vi "MListbox Update Test Step.vi"(8 "error in (no error)":errorcluster, 9 "Rows":string[][](array[string]), 10 "Index":i16=-1, 11 "Multicolumn ListBox in":refnum<class "Multicolumn ListBox.lvclass">) -> (0 "error out":errorcluster, 3 "Multicolumn ListBox out":refnum<class "Multicolumn ListBox.lvclass">)   [LabVIEW 2012, in "Multicolumn ListBox.lvclass"]
uses:
  Multicolumn ListBox.lvclass
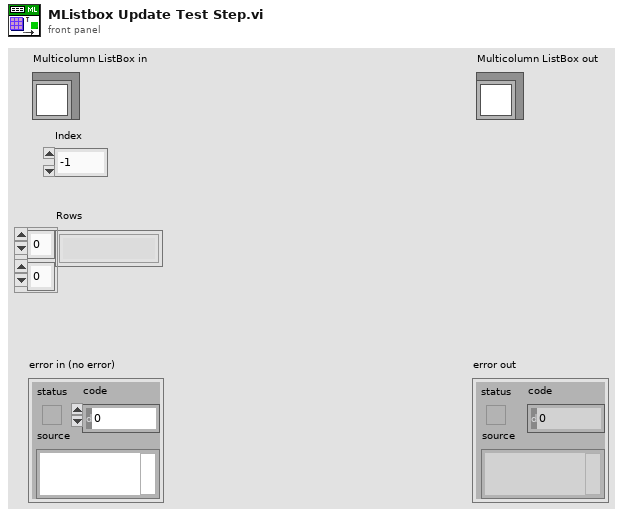
[diagram p1: front panel]
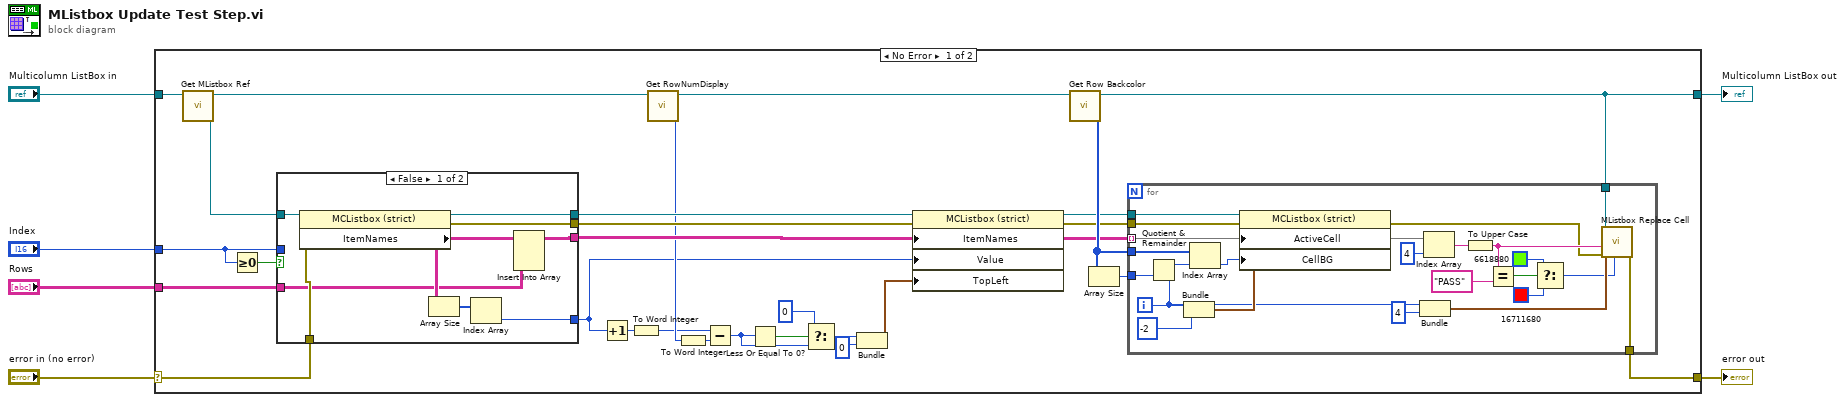
[diagram p0: block diagram]
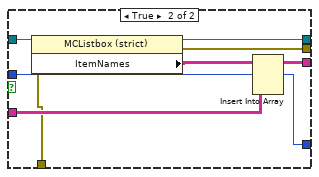
[diagram p2: hidden frame]
diagram:
  n1 = case shown="No Error" "error in (no error)" {
    selector: "error in (no error)" -> [w29 w76]
    tunnel: [w7 w76] -> w5
    tunnel: [w8 w75] -> w3
    tunnel: "Multicolumn ListBox in" -> [w34 w75]
    tunnel: "Index" -> [w19 _]
    tunnel: "Rows" -> [w32 _]
    frame No Error {
      n2 = call "Get MListbox Ref.vi"("Multicolumn ListBox in"=w34) -> ("MListbox Ref"=w33:refnum<vi>, "Multicolumn ListBox out"=w30:refnum<class "Multicolumn ListBox.lvclass">)  [unwired: 8 in, 1 out]
      n3 = Greater Or Equal To 0?(x=w19) -> (x >= 0?=w20:bool)
      n4 = case shown="False" w20 {
        tunnel: w33 -> [w43 w51]
        tunnel: w32 -> [w37 w49]
        tunnel: w29 -> [w41 w48]
        tunnel: [w42 w47] -> w28
        tunnel: [w36 w46] -> w26
        tunnel: [w35 w45] -> w25
        tunnel: w19 -> [_ w44]
        tunnel: [w39 w44] -> w10
        frame False {
          n5 = property class="MCListbox (strict)"(reference=w43, error in=w41) -> (reference out=w42:refnum<vi>, error out=w35:errorcluster, "ItemNames"=w38:string[][])
          n6 = Array Size(array=w38) -> (size(s)=w40:i32[])
          n7 = Index Array(array=w40) -> (element=w39:i32)  [unwired: 1 in]
          n8 = Insert Into Array(array=w38, new element=w37) -> (w36:string[][])  [unwired: 2 in]
        }
        frame True {
          n9 = property class="MCListbox (strict)"(reference=w51, error in=w48) -> (reference out=w47:refnum<vi>, error out=w45:errorcluster, "ItemNames"=w50:string[][])
          n10 = Insert Into Array(array=w50, index (row)=w44, new element=w49) -> (w46:string[][])  [unwired: 1 in]
        }
      }
      n11 = Increment(x=w10) -> (x+1=w21:i32)
      n12 = To Word Integer(number=w21) -> (16bit integer=w9:i16)
      n13 = call "Get RowNumDisplay.vi"("Multicolumn ListBox in"=w30) -> ("RowNumDisplay"=w11:u16, "Multicolumn ListBox out"=w22:refnum<class "Multicolumn ListBox.lvclass">)  [unwired: 8 in, 1 out]
      n14 = To Word Integer(number=w11) -> (16bit integer=w13:i16)
      n15 = Subtract(x=w9, y=w13) -> (x-y=w16:i16)
      n16 = Less Or Equal To 0?(x=w16) -> (x <= 0?=w18:bool)
      n17 = Select(t=0, s=w18, f=w16) -> (s? t:f=w15:i32)
      n18 = Bundle(w15, 0) -> (w12:cluster{i32, i32})  [unwired: 1 in]
      n19 = property class="MCListbox (strict)"(reference=w28, error in=w25, "ItemNames"=w26, "Value"=w10, "TopLeft"=w12) -> (reference out=w27:refnum<vi>, error out=w24:errorcluster)
      n20 = call "Get Row Backcolor.vi"("Multicolumn ListBox in"=w22) -> ("Row Backcolor"=w31:u32[], "Multicolumn ListBox out"=w8:refnum<class "Multicolumn ListBox.lvclass">)  [unwired: 8 in, 1 out]
      n21 = Array Size(array=w31) -> (size(s)=w23:i32)
      n22 = for {
        tunnel: w26 -> [w62] mode=indexing
        tunnel: w27 -> [w71]
        tunnel: w23 -> [w74]
        tunnel: w31 -> [w73]
        tunnel: w24 -> [w68]
        tunnel: w8 -> [w66]
        tunnel: [w52] -> w7
        i -> [w65]
        n23 = Quotient & Remainder(x=w65, y=w74) -> (x-y*floor(x/y)=w72:i32)  [unwired: 1 out]
        n24 = Bundle(w65, "Column"=-2) -> (w69:cluster{i32, "Column":i32})  [unwired: 1 in]
        n25 = Index Array(array=w73, index=w72) -> (element=w67:u32)
        n26 = property class="MCListbox (strict)"(reference=w71, error in=w68, "ActiveCell"=w69, "CellBG"=w67) -> (error out=w53:errorcluster)  [unwired: 1 out]
        n27 = Bundle(w65, "Column"=4) -> (w63:cluster{i32, "Column":i32})  [unwired: 1 in]
        n28 = Index Array(array=w62, index=4) -> (element=w59:string)
        n29 = To Upper Case(1:w59) -> (0:w58:string)
        n30 = Equal?(x=w58, y="PASS") -> (x = y?=w57:bool)
        n31 = Select(t=u32 6618880 ("Backcolor"), s=w57, f=u32 16711680 ("Backcolor")) -> (s? t:f=w54:u32)
        n32 = call "MListbox Replace Cell.vi"("Backcolor"=w54, "error in (no error)"=w53, "String"=w58, "index"=w63, "Multicolumn ListBox in"=w66) -> ("error out"=w52:errorcluster)  [unwired: 5 in, 1 out]
      }
    }
    frame Error {
    }
  }
  "error out" <- w5
  "Multicolumn ListBox out" <- w3
